vi "epx_Vector Diagram Facade.vi"(0 "Data In":T5, 2 "Display State In":T2={"BGColor"=0, "FGColor"=0, "GridColor"=9868950, "Number of Polar Grids"=12, "Number of Circle Grids"=4, "Vector.Active"=0, "Vectors.Properties"=[], "Height"=0, "Width"=0} {"Number of Circle Grids" min=1 max=100 step=1; "Number of Polar Grids" min=1 max=100 step=1}, 3 "Container State":T4) -> (6 "Data Out":T5, 7 "Display State Out":T2={"BGColor"=0, "FGColor"=0, "GridColor"=9868950, "Number of Polar Grids"=12, "Number of Circle Grids"=4, "Vector.Active"=0, "Vectors.Properties"=[], "Height"=0, "Width"=0} {"Number of Circle Grids" min=1 max=100 step=1; "Number of Polar Grids" min=1 max=100 step=1}, 8 "Action":T1)   [LabVIEW 2011, in "NI_EP_Basic.lvlib" / "EPX Vector Diagram.xctl"]
uses:
  <vilib>/addons/Electrical Power/Basic/Controls/Vector Diagram/EPX Vector Diagram.xctl
  <vilib>/addons/Electrical Power/Basic/Controls/Vector Diagram/Abilities/epx_Vector Diagram Data.ctl
  <vilib>/_xctls/Container State.ctl
  <vilib>/addons/Electrical Power/Basic/Controls/Vector Diagram/Abilities/epx_Vector Diagram State.ctl
  <vilib>/addons/Electrical Power/Basic/Controls/Vector Diagram/SubVIs/epx_Vector Type.ctl
  <vilib>/_xctls/Action.ctl
  <vilib>/_xctls/XControlSupport.lvlib
  <vilib>/Utility/miscctls.llb/LVPointTypeDef.ctl
  <vilib>/Utility/miscctls.llb/LVRectTypeDef.ctl
  <vilib>/addons/Electrical Power/Basic/NI_EP_Basic.lvlib
panel:
  out "Vector Diagram":cluster{dbl[], dbl[]}[](graph) caption="Vektorovy graf"
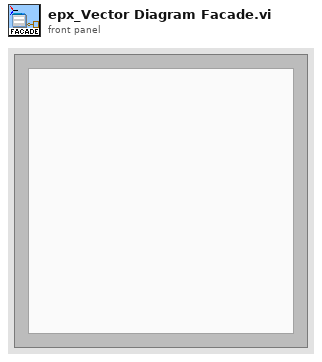
[diagram p1: front panel]
types:
  T1 = typedef "XControlSupport.lvlib/Action.ctl" = cluster{"Data Changed?":bool, "State Changed?":bool, "Action Name":string}
  T2 = typedef "NI_EP_Basic.lvlib/EPX Vector Diagram.xctl/epx_Vector Diagram State.ctl" = cluster{"BGColor":u32, "FGColor":u32, "GridColor":u32, "Number of Polar Grids":i32, "Number of Circle Grids":i32, "Vector.Active":i32, "Vectors.Properties":cluster{"Vector.Type":T3, "Vector.Color":u32, "Vector.Width":u8}[], "Height":u32, "Width":u32}
  T3 = typedef "NI_EP_Basic.lvlib/epx_Vector Type.ctl" = enum16{"Voltage", "Current"}
  T4 = typedef "XControlSupport.lvlib/Container State.ctl" = cluster{"Indicator?":bool, "Run Mode?":bool, " Refnum":refnum<vi>}
  T5 = typedef "NI_EP_Basic.lvlib/EPX Vector Diagram.xctl/epx_Vector Diagram Data.ctl" = cdb[]
  T6 = typedef "LVRectTypeDef.ctl" = cluster{"left":i16, "top":i16, "right":i16, "bottom":i16}
  T7 = typedef "LVPoint32TypeDef.ctl" = cluster{"Horizontal":i32, "Vertical":i32}
  T8 = typedef "LVPointTypeDef.ctl" = cluster{"Horizontal":i16, "Vertical":i16}
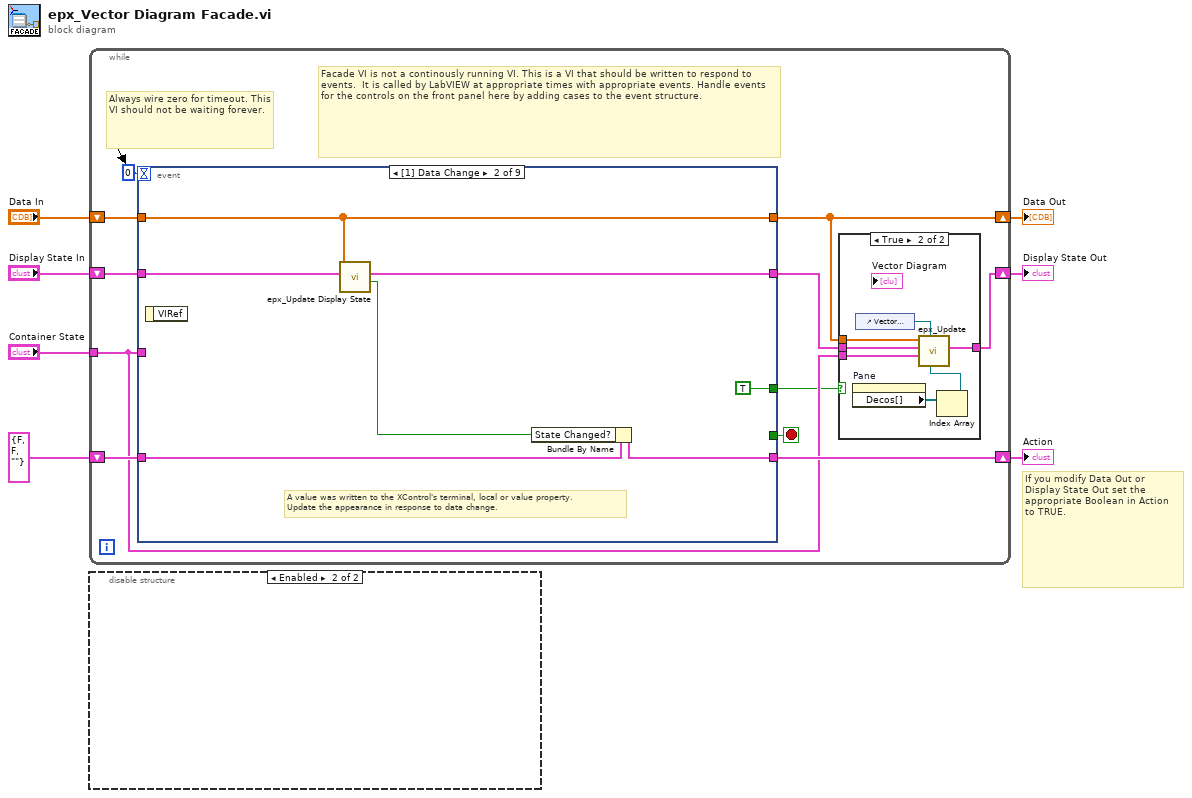
[diagram p0: block diagram]
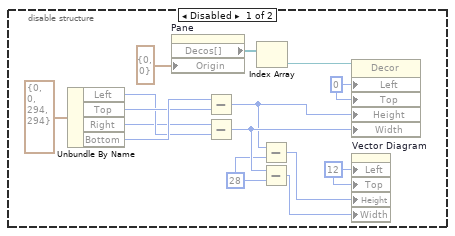
[diagram p2: hidden frame]
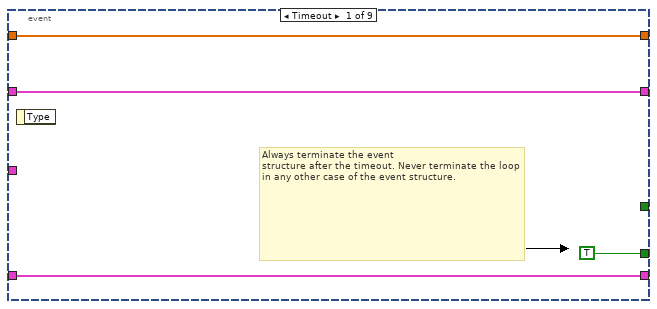
[diagram p4: hidden frame]
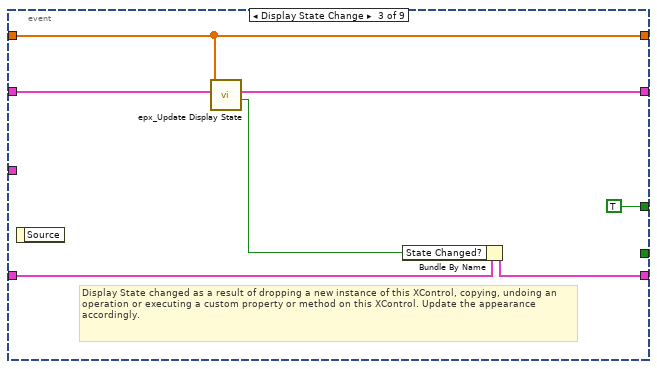
[diagram p5: hidden frame]
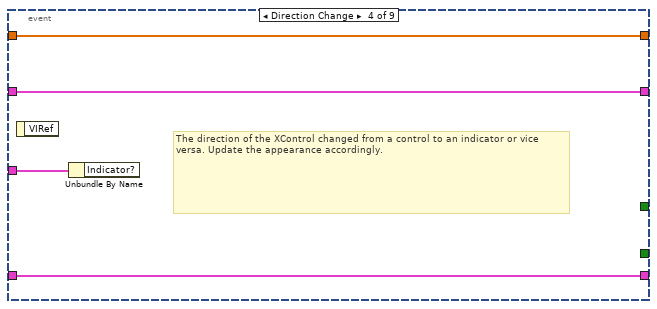
[diagram p6: hidden frame]
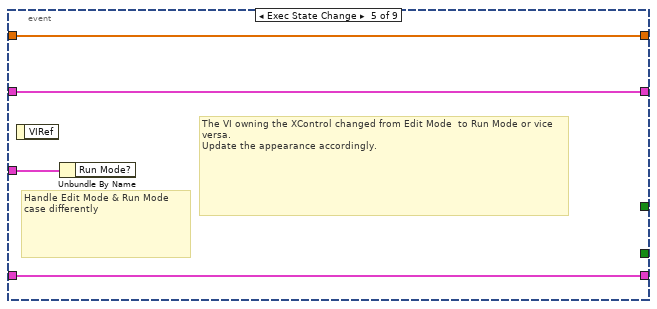
[diagram p7: hidden frame]
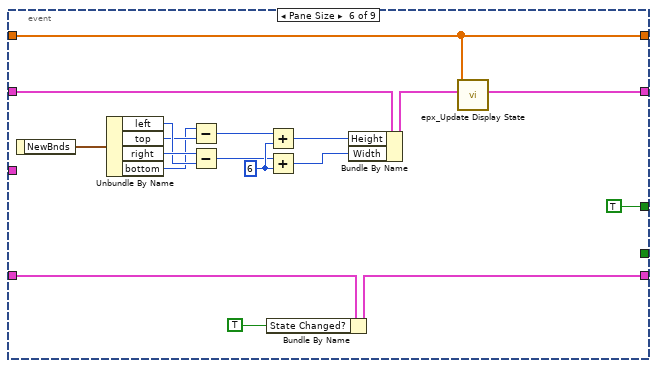
[diagram p8: hidden frame]
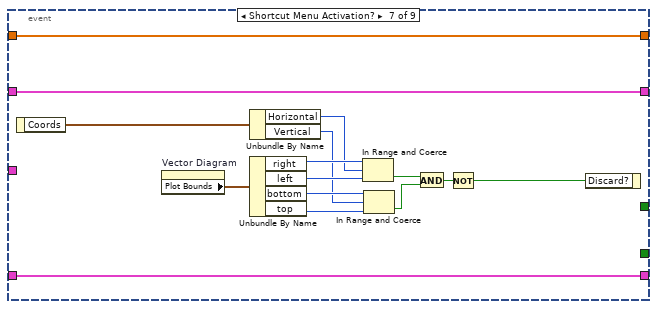
[diagram p9: hidden frame]
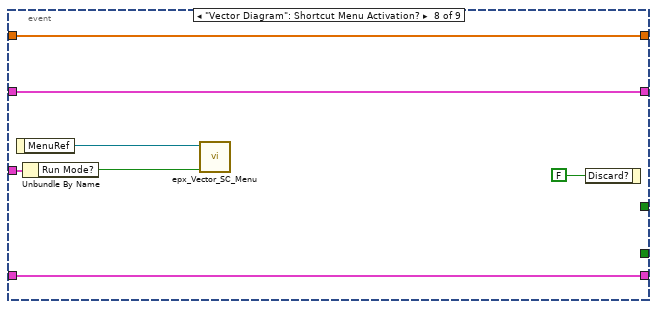
[diagram p10: hidden frame]
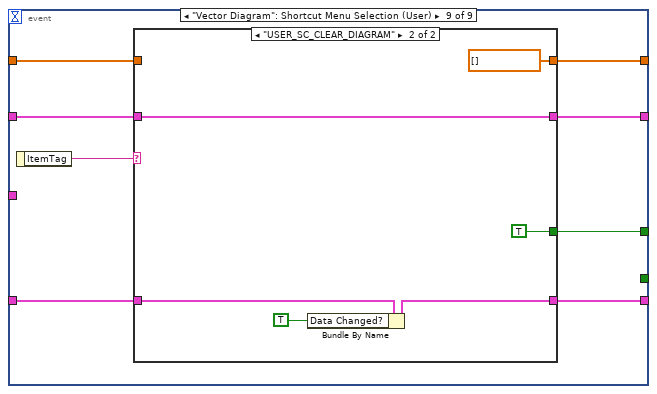
[diagram p11: hidden frame]
diagram:
  # "If you modify Data Out or\nDisplay State Out set the\nappropriate Boolean in Action\nto TRUE."
  n1 = while {
    shift-right: [w8] -> w4
    shift-left: "Display State In" -> [w18]
    tunnel: "Container State" -> [w12]
    shift-right: [w10] -> w7
    shift-left: "Data In" -> [w15]
    shift-right: [w13] -> w2
    shift-left: T1 {"Data Changed?"=FALSE, "State Changed?"=FALSE, "Action Name"=""} ("Action") -> [w14]
    stop <- w17 stop-if-true
    # "Facade VI is not a continously running VI. This is a VI that should be written to respond to events.  It is called by LabVIEW at appropriate times with appropriate events. Handle events for the controls on the front panel here by adding cases to the event structure."
    # "Always wire zero for timeout. This\nVI should not be waiting forever."
    n2 = event shown="[1] Data Change" {
      selector: _ -> [_ _ _ _ _ _ _ _ _]
      dyn-events: _ -> [_ _ _ _ _ _ _ _ _]
      timeout: 0 -> [_ _ _ _ _ _ _ _ _]
      tunnel: w18 -> [w28 w36 w42 w47 w51 w59 w84 w90 w96]
      tunnel: [w28 w35 w41 w47 w51 w53 w84 w90 w97] -> w11
      tunnel: [TRUE _ _ _ _ _ _ _ _] -> w17
      tunnel: w12 -> [_ _ _ w48 w52 _ _ w87 _]
      tunnel: w15 -> [w27 w31 w43 w46 w50 w55 w85 w92 w98]
      tunnel: [w27 w31 w43 w46 w50 w55 w85 w92 w99] -> w10
      tunnel: [w29 w33 w39 w45 w49 w64 w83 w89 w95] -> w13
      tunnel: w14 -> [w29 w34 w40 w45 w49 w65 w83 w89 w94]
      tunnel: [_ TRUE TRUE _ _ TRUE _ _ w93] -> w9
      event Timeout {
        # "Always terminate the event\nstructure after the timeout. Never terminate the loop in any other case of the event structure."
        n3 = event-data() -> ()  [unwired: 1 in, 1 out]
      }
      event Data Change {
        # "A value was written to the XControl's terminal, local or value property.\nUpdate the appearance in response to data change."
        n4 = event-data() -> ()  [unwired: 1 in, 1 out]
        n5 = call <vilib>:"epx_Update Display State.vi"("Display State In"=w36, "Data In"=w31) -> ("State Changed?"=w32:bool, "Display State Out"=w35:T2)  [unwired: 8 in]
        n6 = Bundle By Name(cluster=w34, "State Changed?"=w32) -> (w33:T1)
      }
      event Display State Change {
        # "Display State changed as a result of dropping a new instance of this XControl, copying, undoing an operation or executing a custom property or method on this XControl. Update the appearance accordingly."
        n7 = event-data() -> ()  [unwired: 1 in, 1 out]
        n8 = call <vilib>:"epx_Update Display State.vi"("Display State In"=w42, "Data In"=w43) -> ("State Changed?"=w38:bool, "Display State Out"=w41:T2)  [unwired: 8 in]
        n9 = Bundle By Name(cluster=w40, "State Changed?"=w38) -> (w39:T1)
      }
      event Direction Change {
        # "The direction of the XControl changed from a control to an indicator or vice versa. Update the appearance accordingly."
        n10 = event-data() -> ()  [unwired: 1 in, 1 out]
        n11 = Unbundle By Name(w48) -> ()  [unwired: 1 out]
      }
      event Exec State Change {
        # "The VI owning the XControl changed from Edit Mode  to Run Mode or vice versa.\nUpdate the appearance accordingly."
        # "Handle Edit Mode & Run Mode\ncase differently"
        n12 = event-data() -> ()  [unwired: 1 in, 1 out]
        n13 = Unbundle By Name(w52) -> ()  [unwired: 1 out]
      }
      event Pane Size {
        w61 = i16 6 ("y")
        n14 = event-data() -> ("NewBnds"=w70:T6)  [unwired: 1 in]
        n15 = Unbundle By Name(w70) -> ("left"=w68:i16, "top"=w67:i16, "right"=w69:i16, "bottom"=w66:i16)
        n16 = Subtract(x=w66, y=w67) -> (x-y=w62:i16)
        n17 = Subtract(x=w69, y=w68) -> (x-y=w60:i16)
        n18 = Bundle By Name(cluster=w65, "State Changed?"=TRUE ("Data Changed?")) -> (w64:T1)
        n19 = Add(x=w62, y=w61) -> (x+y=w57:i16)
        n20 = Add(x=w60, y=w61) -> (x+y=w58:i16)
        n21 = Bundle By Name(cluster=w59, "Height"=w57, "Width"=w58) -> (w54:T2)
        n22 = call <vilib>:"epx_Update Display State.vi"("Display State In"=w54, "Data In"=w55) -> ("Display State Out"=w53:T2)  [unwired: 8 in, 1 out]
      }
      event Shortcut Menu Activation? {
        n23 = event-data() -> ("Coords"=w72:T7)  [unwired: 1 in]
        n24 = property on="Vector Diagram" class="XYGraph (strict)"() -> ("Plot Bounds"=w82:T6)  [unwired: 2 in, 2 out]
        n25 = Unbundle By Name(w72) -> ("Horizontal"=w77:i32, "Vertical"=w76:i32)
        n26 = Unbundle By Name(w82) -> ("right"=w80:i16, "left"=w81:i16, "bottom"=w79:i16, "top"=w78:i16)
        n27 = In Range and Coerce(upper limit=w80, x=w77, lower limit=w81) -> (In Range?=w75:bool)  [unwired: 1 out]
        n28 = In Range and Coerce(upper limit=w79, x=w76, lower limit=w78) -> (In Range?=w74:bool)  [unwired: 1 out]
        n29 = And(x=w75, y=w74) -> (x .and. y?=w73:bool)
        n30 = Not(x=w73) -> (.not. x?=w71:bool)
        n31 = event-data("Discard?"=w71) -> ()  [unwired: 1 in, 1 out]
      }
      event "Vector Diagram": Shortcut Menu Activation? {
        n32 = event-data() -> ("MenuRef"=w88:refnum<k9>)  [unwired: 1 in]
        n33 = Unbundle By Name(w87) -> ("Run Mode?"=w86:bool)
        n34 = call <vilib>:"epx_Vector_SC_Menu.vi"("Run Mode?"=w86, "MenuRef"=w88) -> ()  [unwired: 10 in]
        n35 = event-data("Discard?"=FALSE) -> ()  [unwired: 1 in, 1 out]
      }
      event "Vector Diagram": Shortcut Menu Selection (User) {
        n36 = event-data() -> ("ItemTag"=w100:string)  [unwired: 1 in]
        n37 = case shown="\"USER_SC_CLEAR_DIAGRAM\"" w100 {
          tunnel: [w103 T5 [] ("Data In")] -> w99
          tunnel: w98 -> [w103 _]
          tunnel: [w102 w104] -> w97
          tunnel: w96 -> [w102 w104]
          tunnel: [w101 w107] -> w95
          tunnel: w94 -> [w101 w108]
          tunnel: [_ TRUE] -> w93
          frame Default {
          }
          frame "USER_SC_CLEAR_DIAGRAM" {
            n38 = Bundle By Name(cluster=w108, "Data Changed?"=TRUE) -> (w107:T1)
          }
        }
      }
    }
    n39 = case shown="True" w9 {
      tunnel: w12 -> [_ w26]
      tunnel: w11 -> [w19 w25]
      tunnel: w10 -> [_ w24]
      tunnel: [w19 w20] -> w8
      frame False {
      }
      frame True {
        n40 = property on="Pane" class="Pane"() -> ("Decos[]"=w23:refnum<vi>[])  [unwired: 2 in, 2 out]
        n41 = control-ref of="Vector Diagram"() -> (w21:refnum<vi>)
        n42 = Index Array(array=w23) -> (element=w22:refnum<vi>)  [unwired: 1 in]
        n43 = call <vilib>:"epx_Update.vi"("Background Decoratin"=w22, "Vector Diagram"=w21, "Container State"=w26, "Display State In"=w25, "Data In"=w24) -> ("Display State Out"=w20:T2)  [unwired: 5 in, 1 out]
      }
    }
  }
  "Display State Out" <- w4
  "Data Out" <- w7
  "Action" <- w2
  n44 = disable-structure shown="Enabled" {
    frame Disabled {
      w112 = 12 ("Position:Left")
      w111 = i16 28 ("y")
      w116 = 0 ("Position:Left")
      n45 = Unbundle By Name(T6 {"Left"=0, "Top"=0, "Right"=294, "Bottom"=294} ("input cluster")) -> ("Left"=w118:i16, "Top"=w119:i16, "Right"=w117:i16, "Bottom"=w120:i16)
      n46 = property on="Pane" class="Pane"("Origin"=T8 {"Horizontal"=0, "Vertical"=0}) -> ("Decos[]"=w114:refnum<vi>[])  [unwired: 2 in, 2 out]
      n47 = Subtract(x=w120, y=w119) -> (x-y=w121:i16)
      n48 = Subtract(x=w117, y=w118) -> (x-y=w123:i16)
      n49 = Index Array(array=w114) -> (element=w115:refnum<vi>)  [unwired: 1 in]
      n50 = Subtract(x=w121, y=w111) -> (x-y=w122:i16)
      n51 = Subtract(x=w123, y=w111) -> (x-y=w124:i16)
      n52 = property class="Decor"(reference=w115, "Left"=w116, "Top"=w116, "Height"=w121, "Width"=w123) -> ()  [unwired: 1 in, 2 out]
      n53 = property on="Vector Diagram" class="XYGraph (strict)"("Left"=w112, "Top"=w112, "Height"=w122, "Width"=w124) -> ()  [unwired: 2 in, 2 out]
    }
    frame Enabled {
    }
  }
